vi "Setup.vi"(8 "error in (no error)":errorcluster, 9 "Str Refnum":refnum<vi>, 10 "VI Reference":refnum<vi>, 11 "Msg_Error in":refnum<class "ListSelection.lvclass">) -> (0 "error out":errorcluster, 2 "VI reference (dup)":refnum<vi>, 3 "Msg_Error out":refnum<class "ListSelection.lvclass">)   [LabVIEW 2012, in "ListSelection.lvlib" / "ListSelection.lvclass"]
uses:
  ListSelection.lvclass
  ListSelection.lvclass/ListSelection.ctl
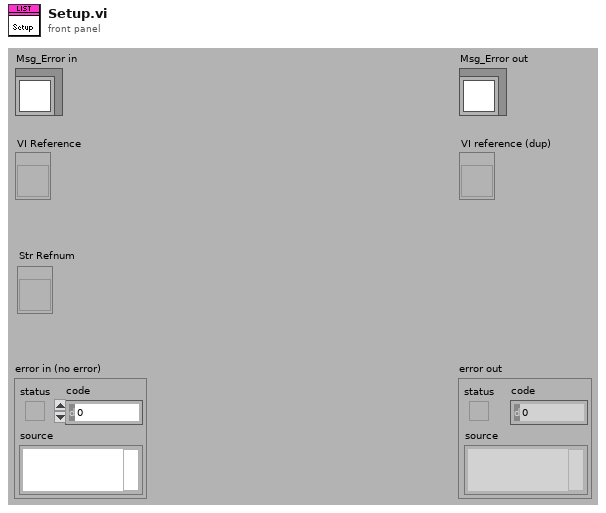
[diagram p1: front panel]
types:
  T1 = typedef "ListSelection.lvlib/ListSelection.lvclass/Selection Mode.ctl" = enum16{"Zero or one", "One", "Zero or more", "One or more"}
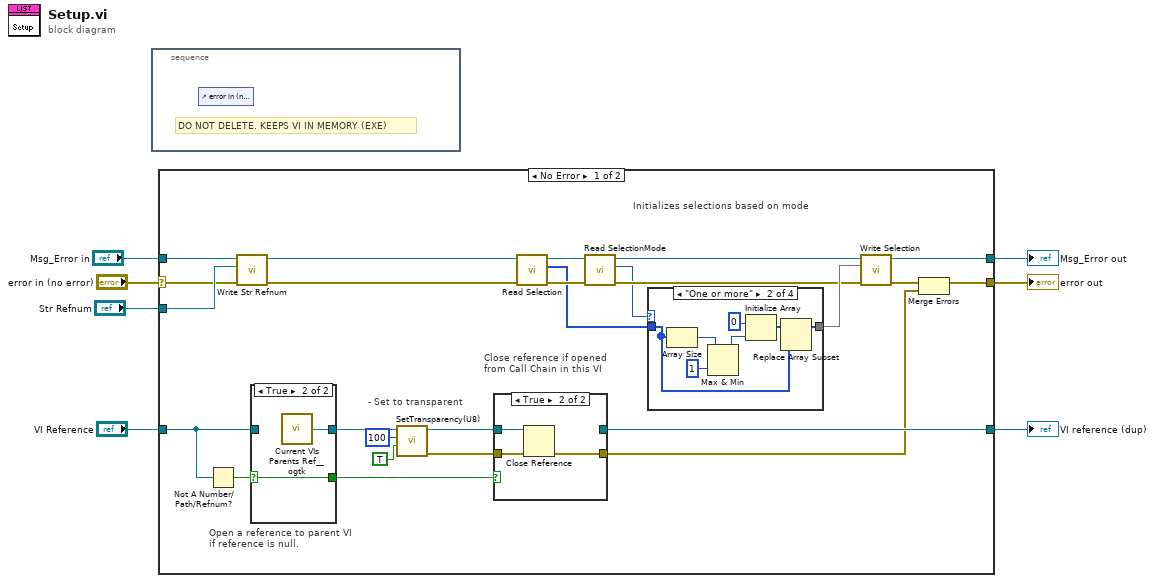
[diagram p0: block diagram]
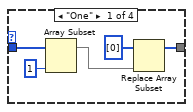
[diagram p2: hidden frame]
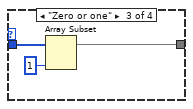
[diagram p3: hidden frame]
diagram:
  n1 = stacked-sequence {
    frame #0 {
      # "DO NOT DELETE. KEEPS VI IN MEMORY (EXE)"
      n2 = control-ref of="error in (no error)"() -> ()  [unwired: 1 out]
    }
  }
  n3 = case shown="No Error" "error in (no error)" {
    selector: "error in (no error)" -> [w23 w60]
    tunnel: [w11 w60] -> w4
    tunnel: [w22 w59] -> w5
    tunnel: "Msg_Error in" -> [w24 w59]
    tunnel: "VI Reference" -> [w13 w58]
    tunnel: [w28 w58] -> w3
    tunnel: "Str Refnum" -> [w25 _]
    frame No Error {
      # "Open a reference to parent VI\nif reference is null."
      # "Close reference if opened\nfrom Call Chain in this VI"
      # "Initializes selections based on mode"
      # "- Set to transparent"
      n4 = Not A Number/Path/Refnum?(number/path/refnum=w13) -> (NaN/Path/Refnum?=w31:bool)
      n5 = call-dynamic "Write Str Refnum.vi"("error in (no error)"=w23, "Str Refnum"=w25, "Dialog.lvclass in"=w24) -> ("error out"=w8:errorcluster, "Dialog.lvclass out"=w9:refnum<class "ListSelection.lvclass">)  [unwired: 7 out]
      n6 = case shown="True" w31 {
        selector: w31 -> [w54 w56]
        tunnel: w13 -> [w55 _]
        tunnel: [w55 w57] -> w30
        tunnel: [w54 w56] -> w29
        frame False {
        }
        frame True {
          n7 = call <userlib>:"Current VIs Parents Ref__ogtk.vi"() -> ("Calling VI's Reference"=w57:refnum<vi>)  [unwired: 2 out]
        }
      }
      n8 = call "SetTransparency(U8).vi"("Run VI Transparently (T)"=TRUE, "Transparency (%)"=u8 100, "VI Reference (calling VI)"=w30) -> ("error out"=w14:errorcluster, "dup VI Reference"=w26:refnum<vi>)  [unwired: 1 in, 6 out]
      n9 = case shown="True" w29 {
        tunnel: w26 -> [w50 w53]
        tunnel: [w50 _] -> w28
        tunnel: w14 -> [w49 w52]
        tunnel: [w49 w51] -> w10
        frame False {
        }
        frame True {
          n10 = Close Reference(reference=w53, error in (no error)=w52) -> (error out=w51:errorcluster)
        }
      }
      n11 = call "Read Selection.vi"("error in (no error)"=w8, "ListSelection in"=w9) -> ("error out"=w20:errorcluster, "Selection"=w18:i32[], "ListSelection out"=w21:refnum<class "ListSelection.lvclass">)  [unwired: 7 in]
      n12 = call-dynamic "Read SelectionMode.vi"("error in (no error)"=w20, "Msg_Error.lvclass in"=w21) -> ("error out"=w16:errorcluster, "Selection Mode"=w15:T1, "Msg_Error.lvclass out"=w19:refnum<class "ListSelection.lvclass">)  [unwired: 7 in]
      n13 = case shown="\"One or more\"" w15 {
        tunnel: w18 -> [w37 w42 w47 w48]
        tunnel: [w33 w44 w45 w48] -> w17
        frame "One" {
          n14 = Array Subset(array=w37, length=1) -> (w34:i32[])  [unwired: 1 in]
          n15 = Replace Array Subset(array=i32[] [0] ("Selection"), new element=w34) -> (w33:i32[])  [unwired: 1 in]
        }
        frame "One or more" {
          n16 = Array Size(array=w42) -> (size(s)=w39:i32)
          n17 = Max & Min(x=w39, y=1) -> (max(x,y)=w38:i32)  [unwired: 1 out]
          n18 = Initialize Array(0 ("Numeric"), w38) -> (w43:i32[])
          n19 = Replace Array Subset(array=w43, new element=w42) -> (w44:i32[])  [unwired: 1 in]
        }
        frame "Zero or one" {
          n20 = Array Subset(array=w47, length=1) -> (w45:i32[])  [unwired: 1 in]
        }
        frame "Zero or more" {
        }
      }
      n21 = call "Write Selection.vi"("error in (no error)"=w16, "Selection"=w17, "ListSelection in"=w19) -> ("error out"=w12:errorcluster, "ListSelection out"=w22:refnum<class "ListSelection.lvclass">)  [unwired: 7 in]
      n22 = Merge Errors(w12, w10) -> (w11:errorcluster)
    }
    frame Error {
    }
  }
  "error out" <- w4
  "Msg_Error out" <- w5
  "VI reference (dup)" <- w3
